vi "CmdSetOman_ParseProg.vi"(5 "progress":string) -> (1 "tot sequence":i32, 2 "imnumber":i32, 3 "imagenumber":i32, 4 "read prog":i32, 6 "exp prog":dbl, 8 "write prog":i32, 10 "detstatus":string, 12 "imstatus":string, 13 "imagepath":string, 14 "imagename":string)   [LabVIEW 2016]
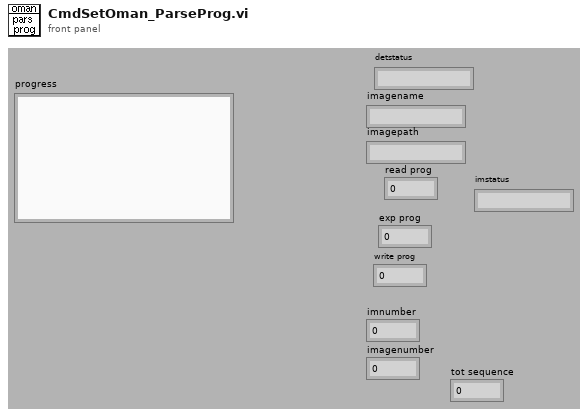
[diagram p1: front panel]
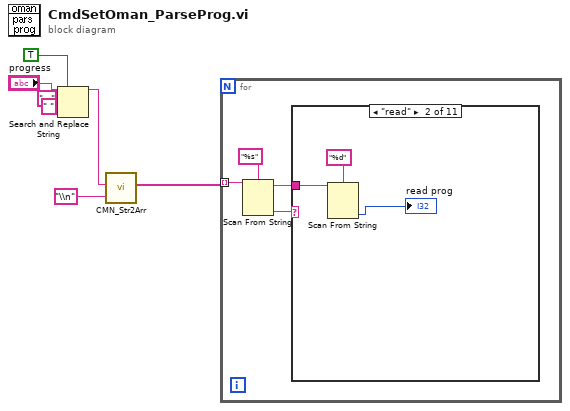
[diagram p0: block diagram]
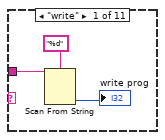
[diagram p2: hidden frame]
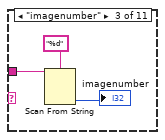
[diagram p3: hidden frame]
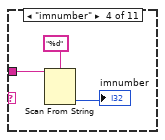
[diagram p4: hidden frame]
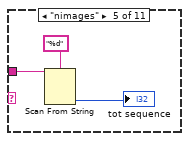
[diagram p5: hidden frame]
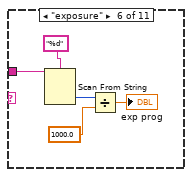
[diagram p6: hidden frame]
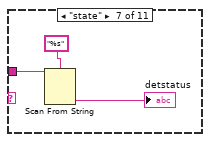
[diagram p7: hidden frame]
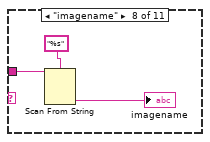
[diagram p8: hidden frame]
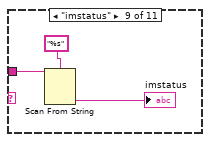
[diagram p9: hidden frame]
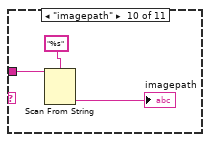
[diagram p10: hidden frame]
diagram:
  n1 = Search and Replace String(replace all?=TRUE ("replace all? (F)"), input string="progress", search string="=", replace string=" " ("replace string (\"\")")) -> (result string=w3:string)  [unwired: 1 in, 6 out]
  n2 = call "CMN_Str2Arr.vi"("separator"="\\n", "string in"=w3) -> ("Array out"=w1:string[])  [unwired: 2 in, 7 out]
  n3 = for {
    tunnel: w1 -> [w11] mode=indexing
    n4 = Scan From String(format string="%s", input string=w11) -> (remaining string=w8:string, output 1=w9:string)  [unwired: 2 in, 3 out]
    n5 = case shown="\"read\"" w9 {
      tunnel: w8 -> [w14 w17 w20 w23 w26 w31 w34 w37 w40 w43 _]
      frame "write" {
        n6 = Scan From String(format string="%d", input string=w14) -> (output 1=→"write prog":i32)  [unwired: 2 in, 4 out]
      }
      frame "read" {
        n7 = Scan From String(format string="%d", input string=w17) -> (output 1=→"read prog":i32)  [unwired: 2 in, 4 out]
      }
      frame "imagenumber" {
        n8 = Scan From String(format string="%d", input string=w20) -> (output 1=→"imagenumber":i32)  [unwired: 2 in, 4 out]
      }
      frame "imnumber" {
        n9 = Scan From String(format string="%d", input string=w23) -> (output 1=→"imnumber":i32)  [unwired: 2 in, 4 out]
      }
      frame "nimages" {
        n10 = Scan From String(format string="%d", input string=w26) -> (output 1=→"tot sequence":i32)  [unwired: 2 in, 4 out]
      }
      frame "exposure" {
        n11 = Scan From String(format string="%d", input string=w31) -> (output 1=w29:i32)  [unwired: 2 in, 4 out]
        n12 = Divide(x=w29, y=1000.0) -> (x/y=→"exp prog":dbl)
      }
      frame "state" {
        n13 = Scan From String(format string="%s", input string=w34) -> (output 1=→"detstatus":string)  [unwired: 2 in, 4 out]
      }
      frame "imagename" {
        n14 = Scan From String(format string="%s", input string=w37) -> (output 1=→"imagename":string)  [unwired: 2 in, 4 out]
      }
      frame "imstatus" {
        n15 = Scan From String(format string="%s", input string=w40) -> (output 1=→"imstatus":string)  [unwired: 2 in, 4 out]
      }
      frame "imagepath" {
        n16 = Scan From String(format string="%s", input string=w43) -> (output 1=→"imagepath":string)  [unwired: 2 in, 4 out]
      }
      frame Default {
      }
    }
  }
